vi "纳清DO电极校准.vi"() -> ()   [LabVIEW 2016, in "斯坦道多参数.lvlib"]
uses:
  <vilib>/Utility/miscctls.llb/LVPointTypeDef.ctl
  <vilib>/Analysis/NI_AALBase.lvlib
panel:
  out "标液2":string="饱和标准液"
  out "标液1":string="零点标准液"
  out "第二点信号值":dbl
  out "第一点信号值":dbl
  out "盐度":sgl format="%#.2f"
  out "大气压力":sgl format="%#.2f"
  out "饱和值":sgl format="%#.2f"
  out "报警信息":string
  out "通讯状态":string
  out "第二点校准值":dbl
  out "第一点校准值":dbl
  in  "校准停止":bool
  in  "校准启动":bool
  in  "校准模式":enum16{"两点校准", "单点校准"}(ring)=enum."单点校准"
  out "最小值":sgl format="%#.2f"
  out "最大值":sgl format="%#.2f"
  out "波形图表":sgl(graph) caption="历史曲线"
  out "mean":dbl caption="均值" format="%#.2f"
  out "standard deviation":dbl caption="标准差" format="%#.2f"
  out "变异系数":dbl format="%#.6f"
  out "测量值":sgl format="%#.2f"
  out "提示":string
  out "原始光强数值":sgl caption="信号值" format="%#.6f"
  out "温度":dbl format="%#.2f"
  # "DO电极设定"
  # "℃"
  # "mg/L"
  # "%"
  # "nA"
  # "kPa"
  # "ppt"
  # "请选择校准模式:"
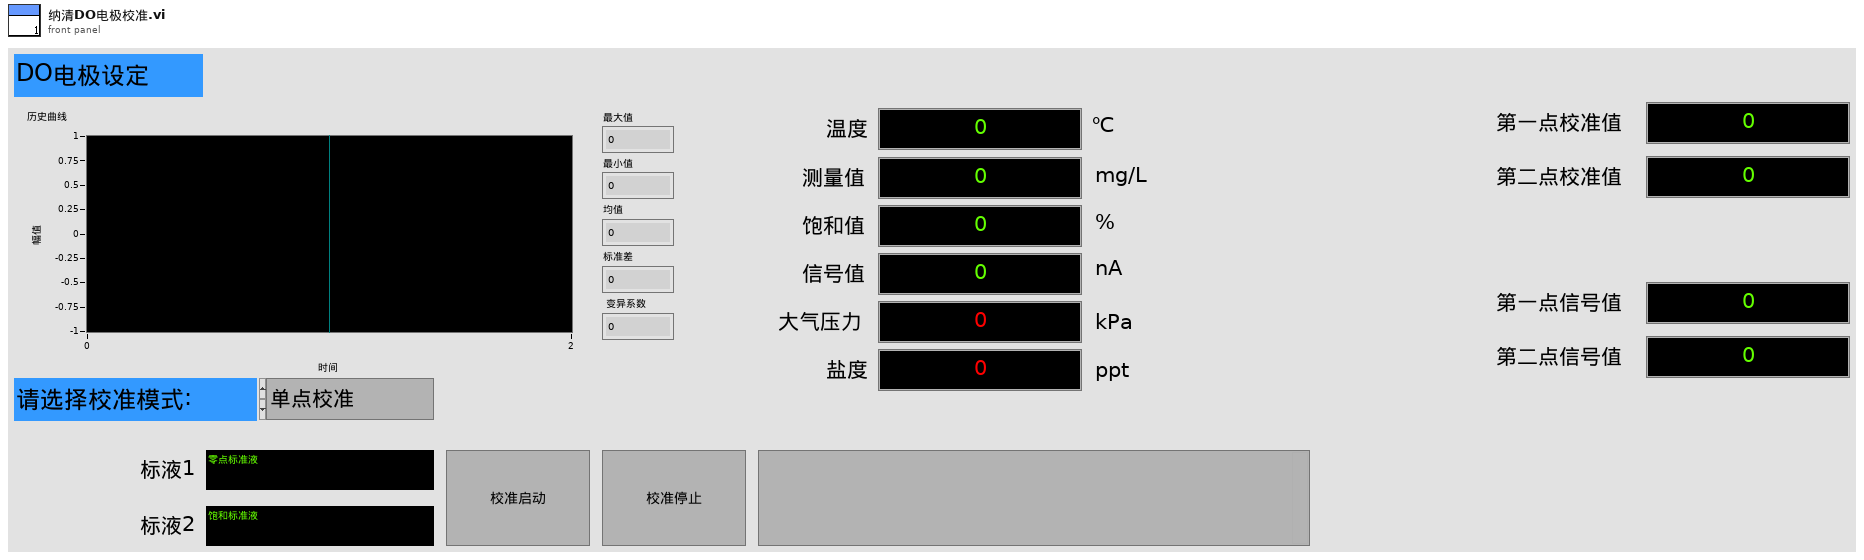
[diagram p1: front panel]
types:
  T1 = typedef "LVPointTypeDef.ctl" = cluster{"Horizontal":i16, "Vertical":i16}
  T2 = cluster{"报警码":u16, "溶解氧数值（mg/L）":sgl, "溶解氧数据（%）":sgl, "温度数据":sgl, "溶解氧原始信号 nA":sgl, "大气压力":sgl, "盐度":sgl, "0X0009_NC":string, "产品名称":string, "序列号":string, "硬件版本":string, "软件版本":string, "通讯地址":u16, "波特率":u16, "设备类型":u16, "0X0026_NC":string, "第一点原始数据":sgl, "第一点校准数据":sgl, "第二点原始数据":sgl, "第二点校准数据":sgl, "探头校准命令":u16, "温度校准参数":sgl, "温度校准命令":u16}
  T3 = enum8{"Enabled", "Disabled", "Disabled and Grayed Out"}
  T4 = cluster{"报警码":u16, "溶解氧数值（mg/L）":sgl, "溶解氧数据（%）":sgl, "温度数据":sgl, "溶解氧原始信号 nA":sgl, "大气压力":sgl, "盐度":sgl, "0X0009_NC":string, "产品名称":string, "序列号":string, "硬件版本":string, "软件版本":string, "通讯地址":u16, "波特率":u16, "设备类型":u16, "0X0026_NC":string, "第一点原始数据":sgl, "0X0033 NC":sgl, "第二点原始数据":sgl, "0X0037 NC":sgl, "探头校准命令":u16, "温度校准参数":sgl, "温度校准命令":u16}
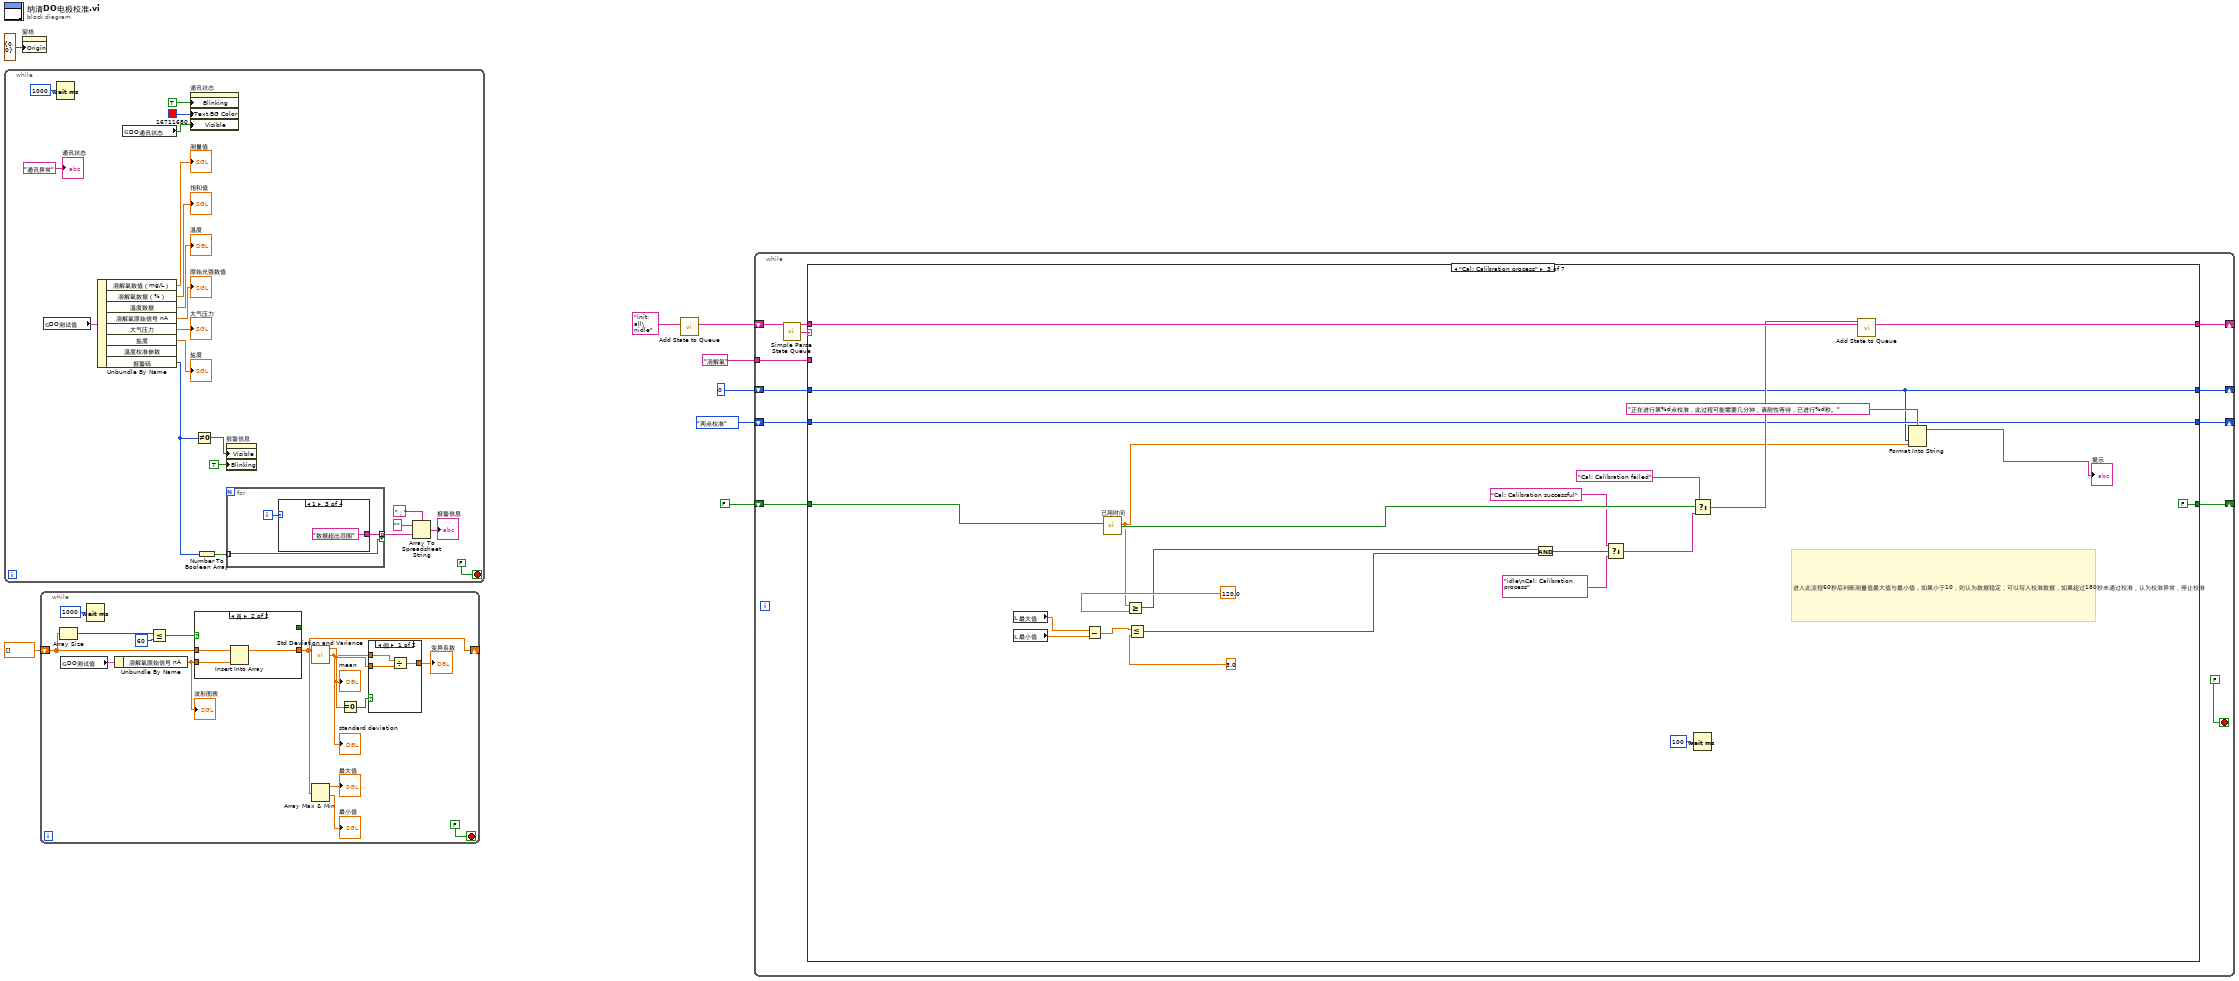
[diagram p0: block diagram]
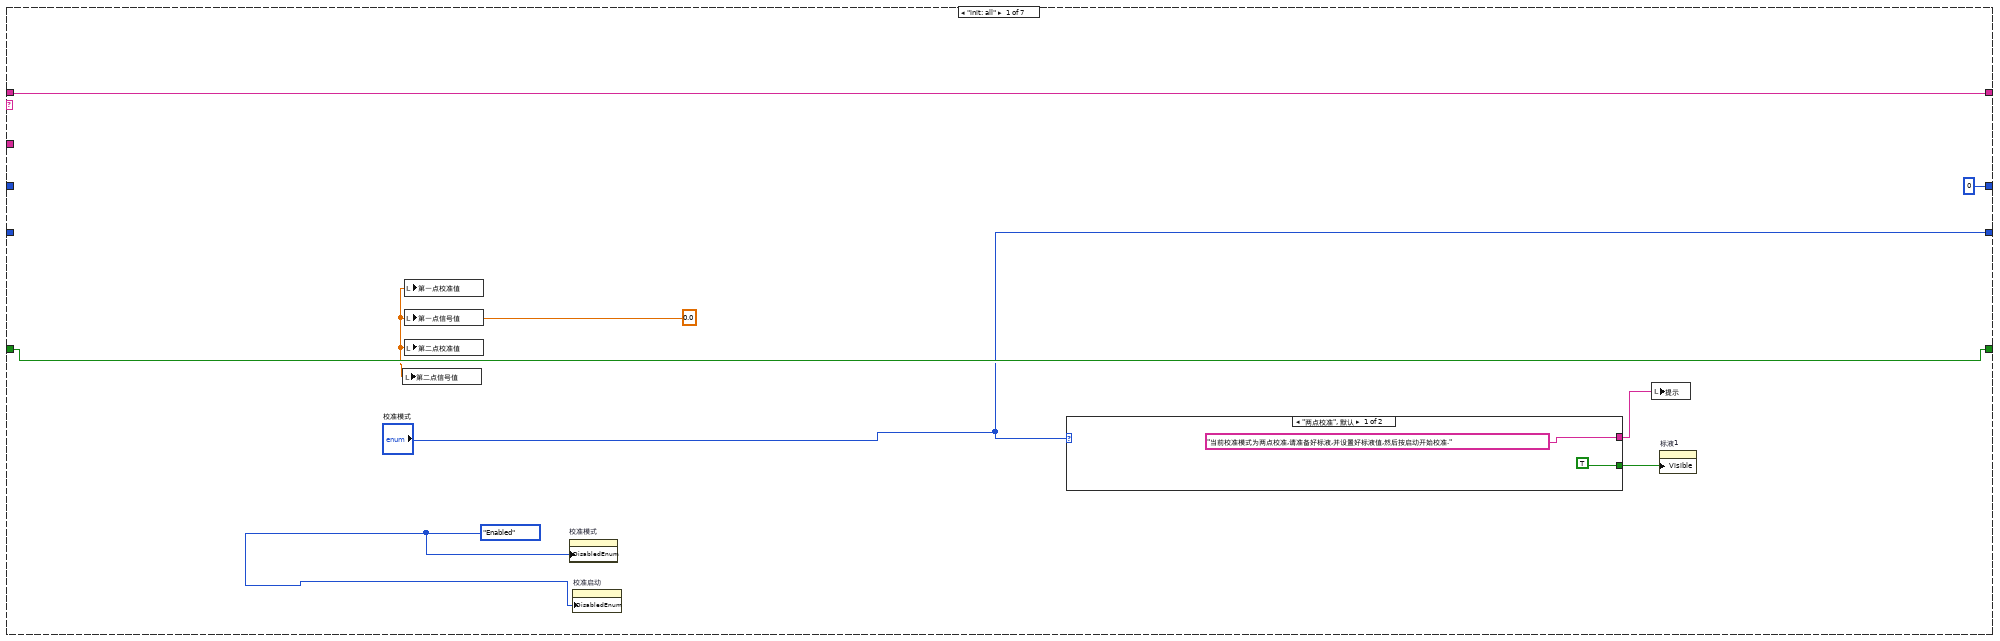
[diagram p2: hidden frame]
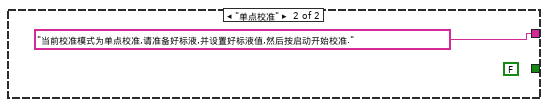
[diagram p3: hidden frame]
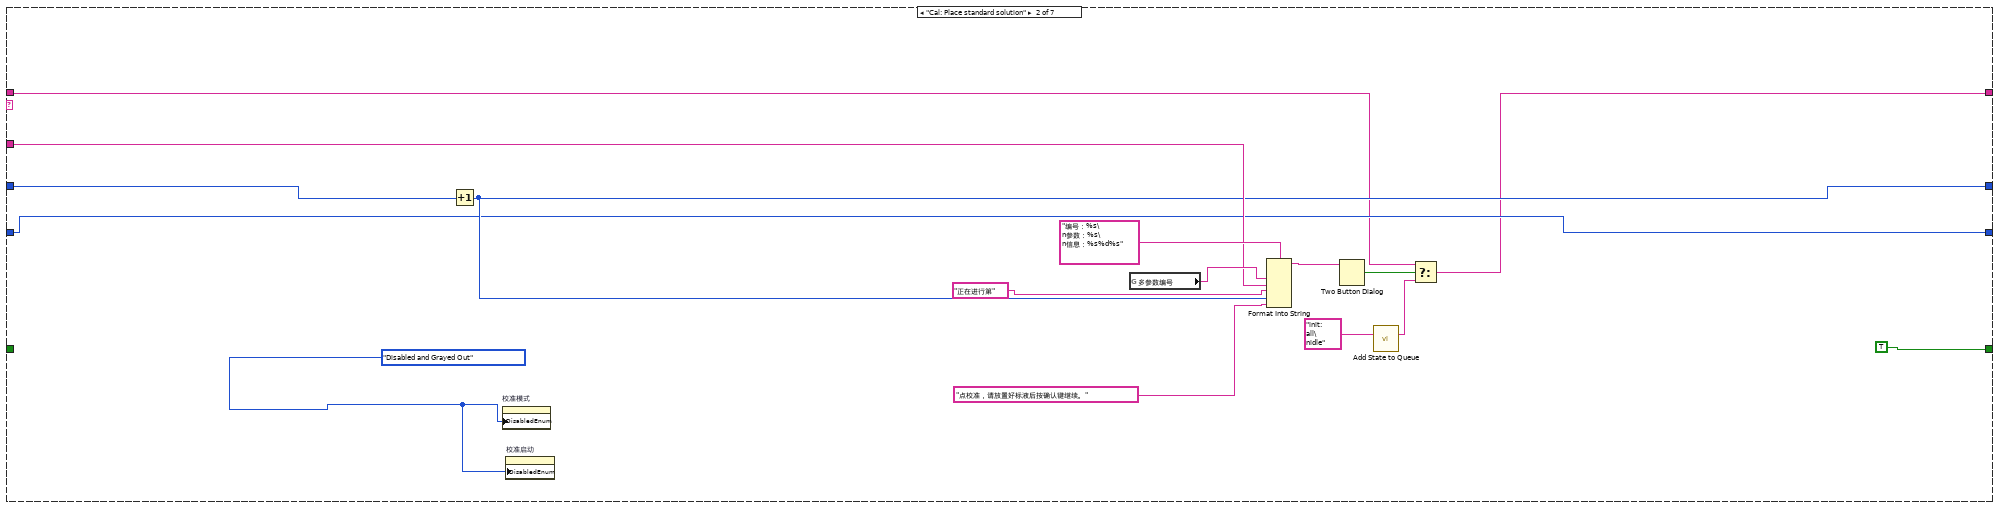
[diagram p4: hidden frame]
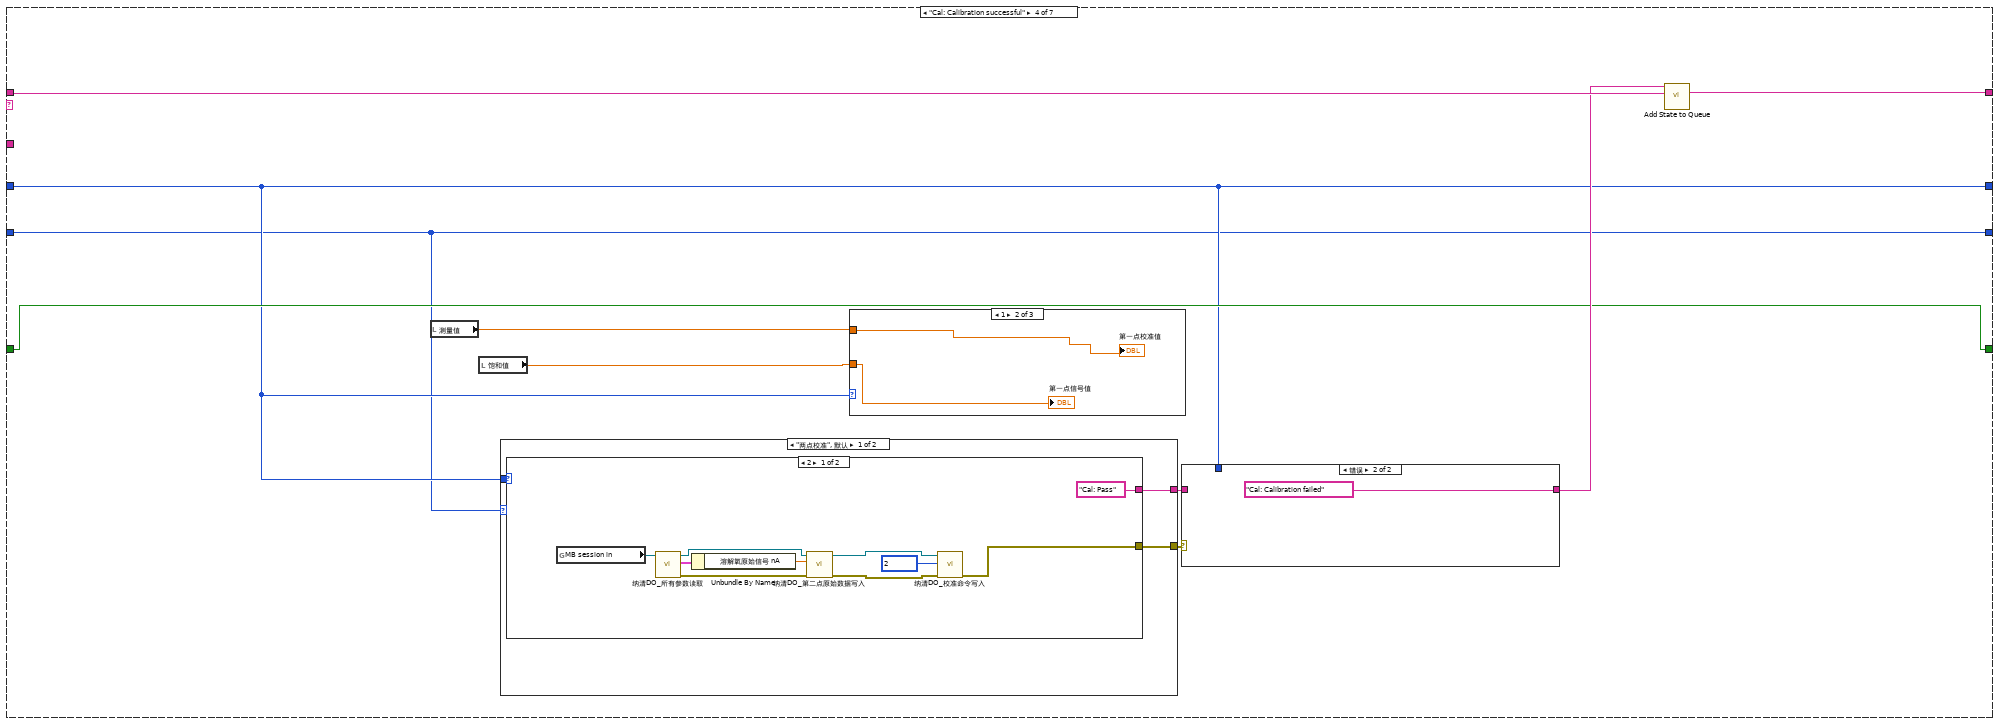
[diagram p5: hidden frame]
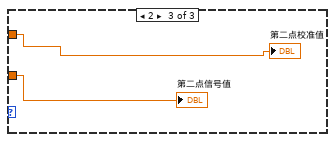
[diagram p7: hidden frame]
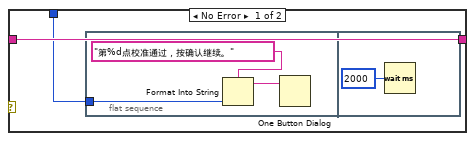
[diagram p8: hidden frame]
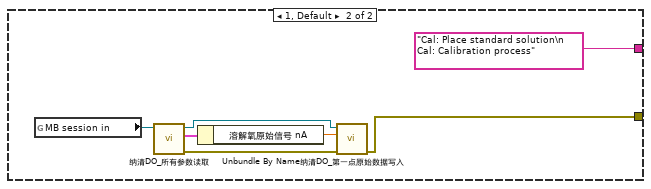
[diagram p9: hidden frame]
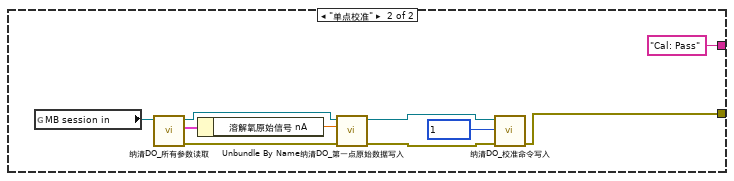
[diagram p10: hidden frame]
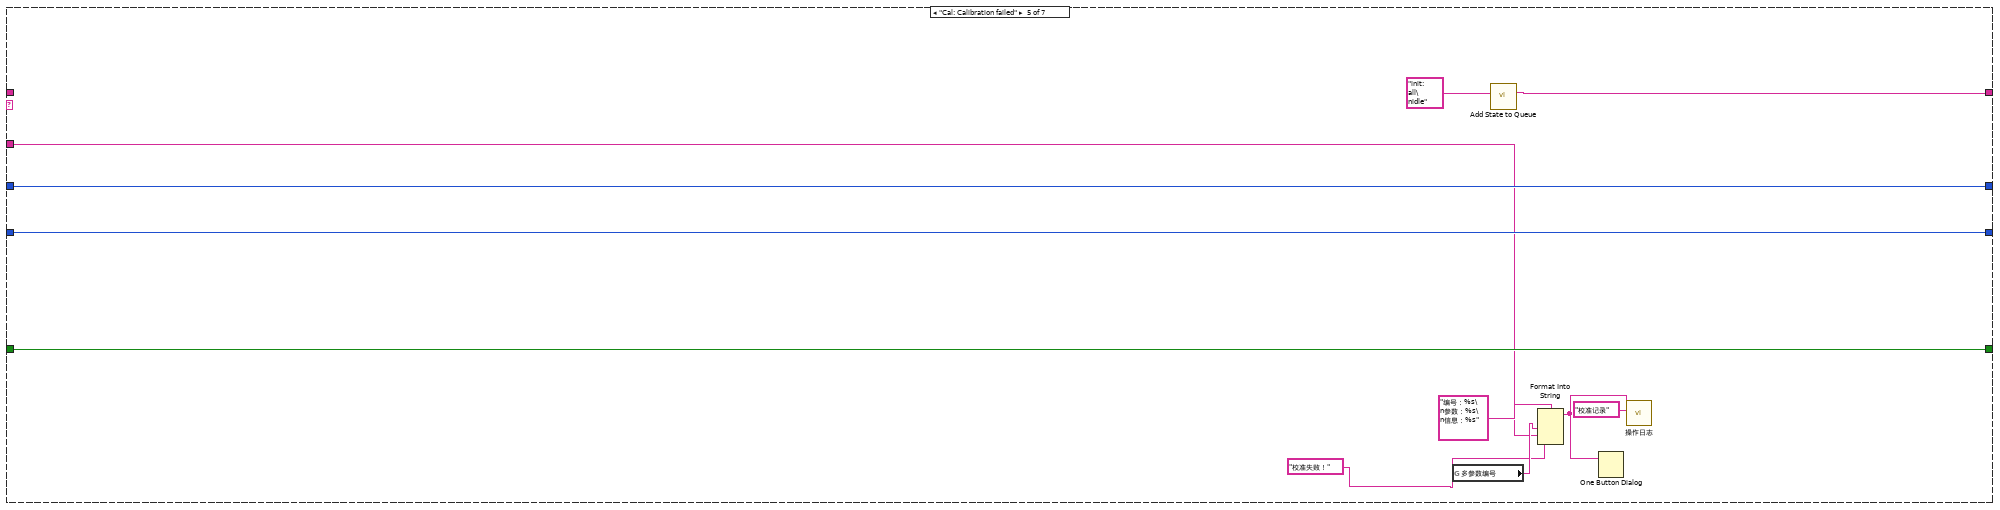
[diagram p11: hidden frame]
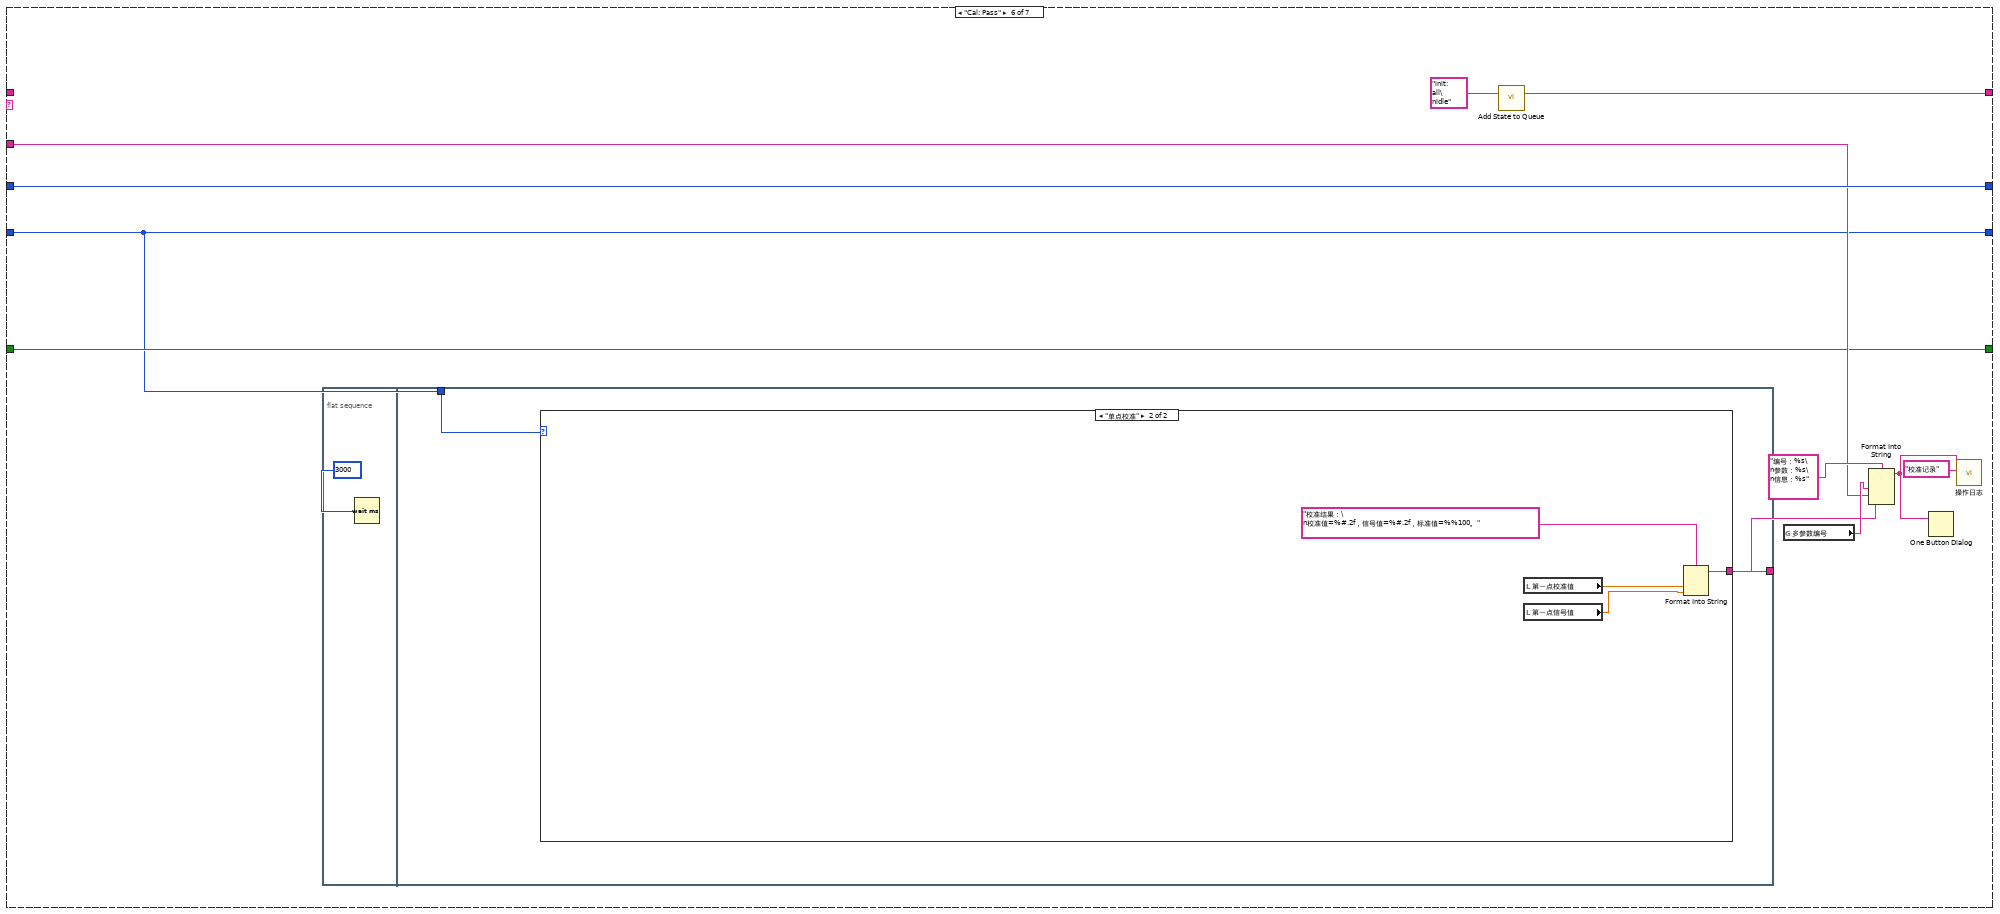
[diagram p12: hidden frame]
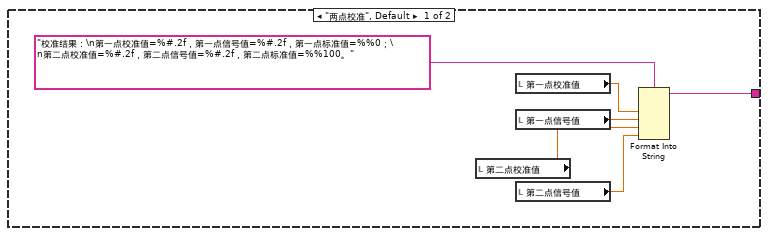
[diagram p13: hidden frame]
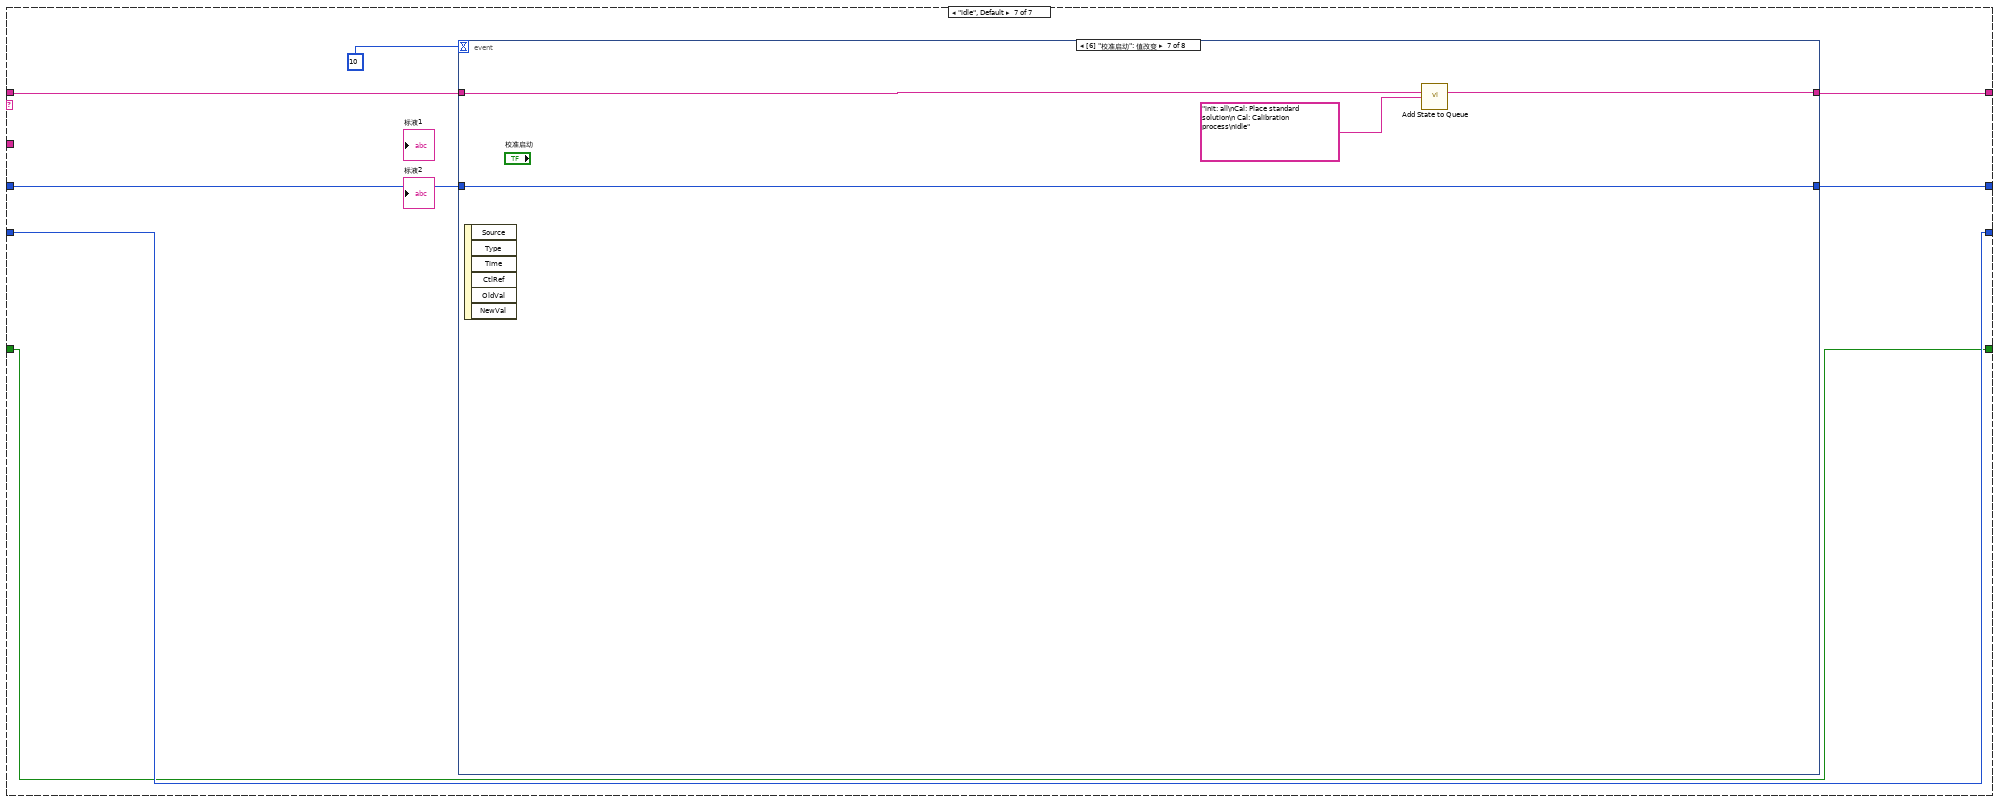
[diagram p14: hidden frame]
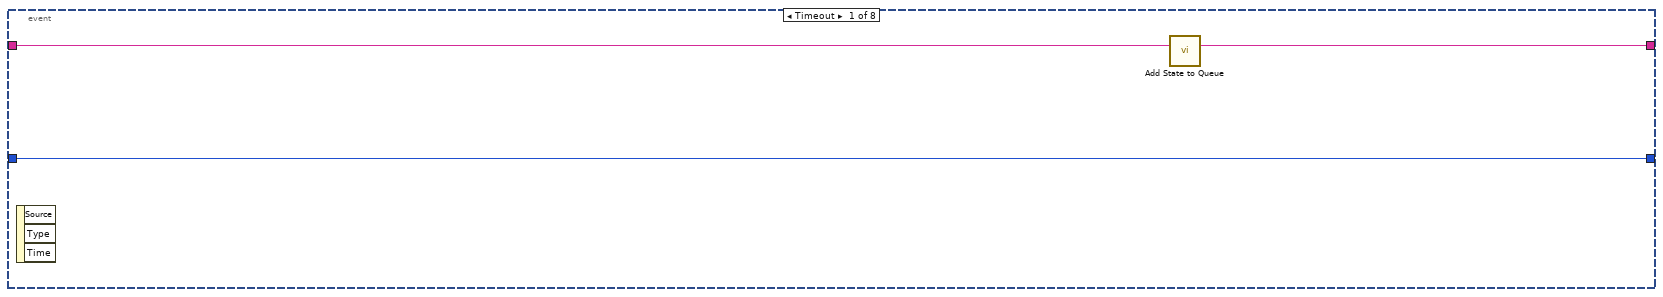
[diagram p15: hidden frame]
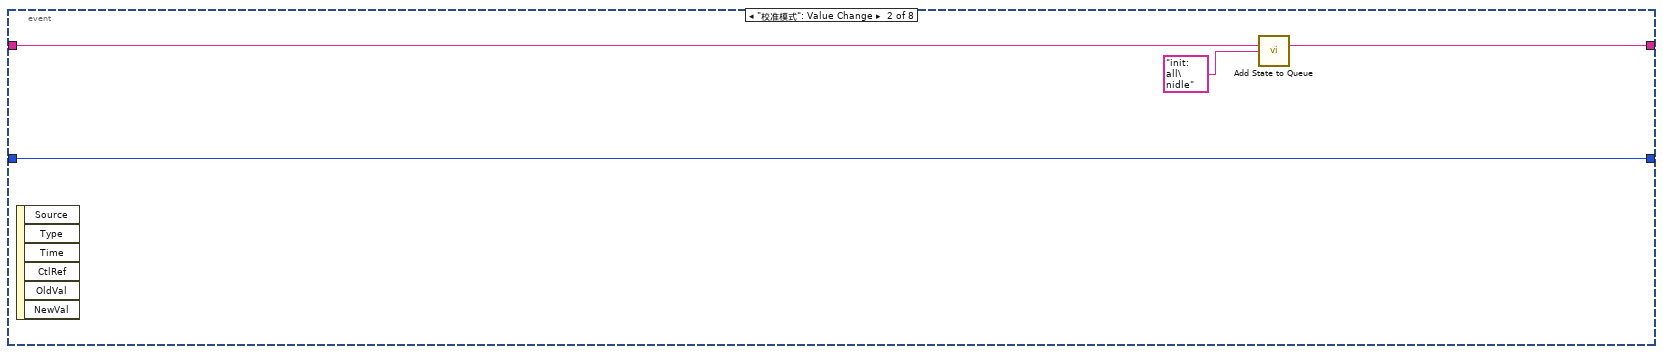
[diagram p16: hidden frame]
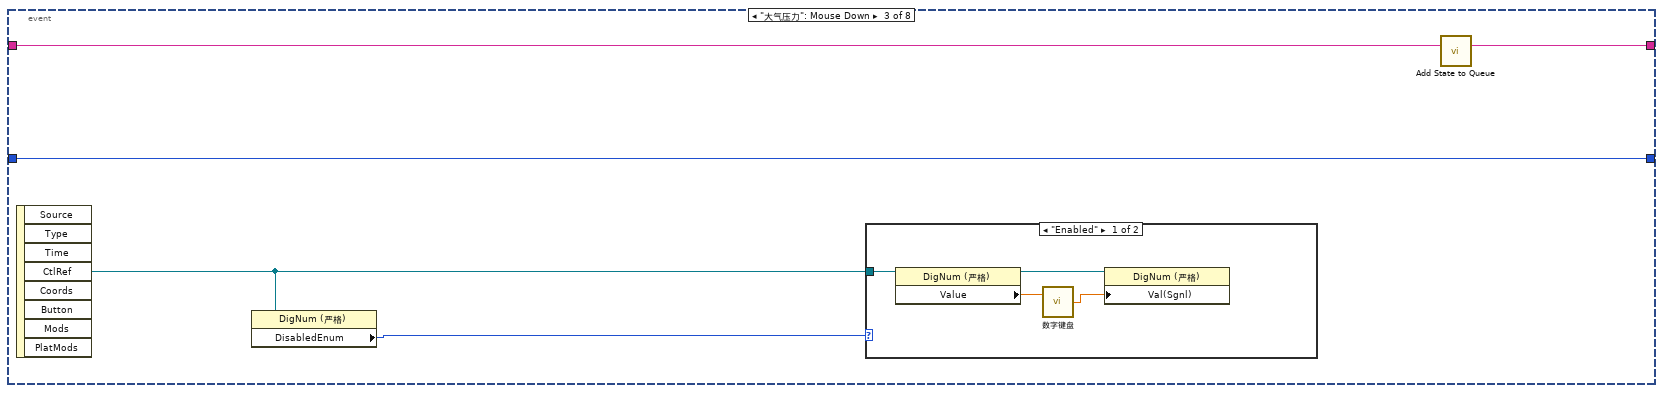
[diagram p17: hidden frame]
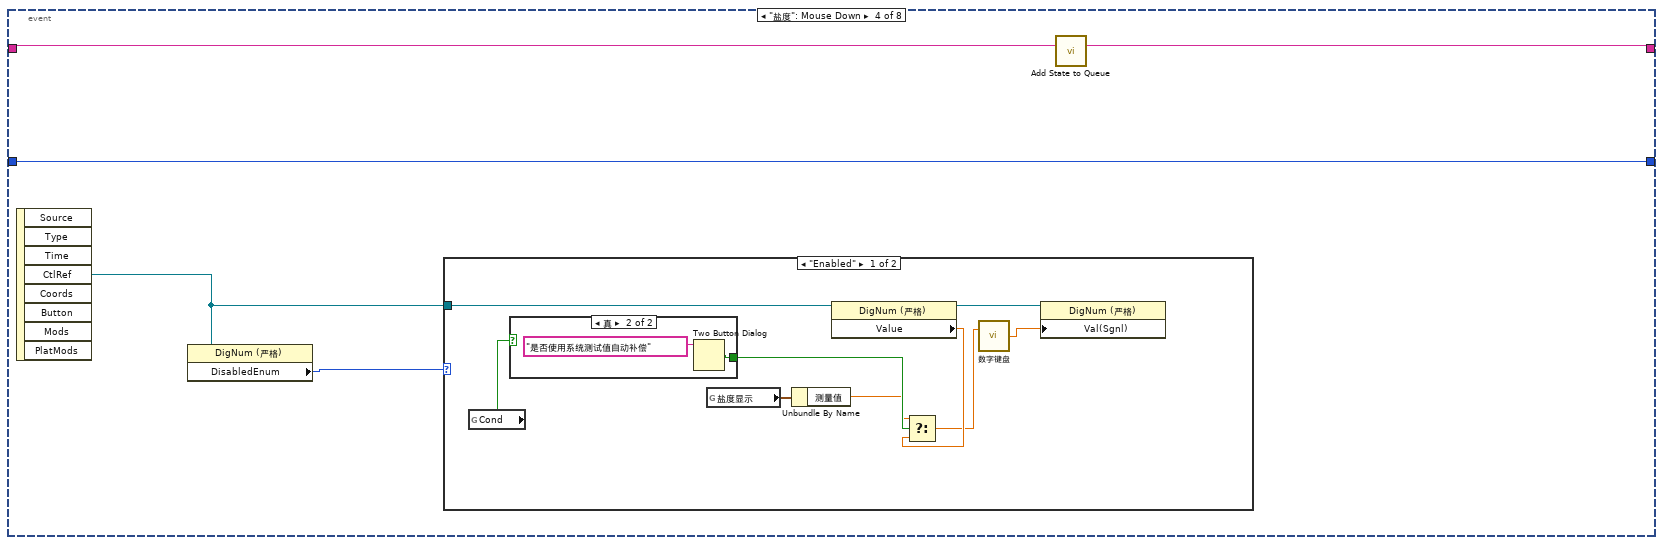
[diagram p19: hidden frame]
diagram:
  n1 = while {
    stop <- FALSE stop-if-true
    n2 = global read "纳清过程全局变量.vi" "DO测试值"() -> (w27:T2)
    n3 = Wait (ms)(milliseconds to wait=u32 1000 ("等待时间（毫秒）")) -> ()  [unwired: 1 out]
    n4 = Unbundle By Name(w27) -> ("溶解氧数值（mg/L）"=→"测量值":sgl, "溶解氧数据（%）"=→"饱和值":sgl, "温度数据"=→"温度":sgl, "溶解氧原始信号 nA"=→"原始光强数值":sgl, "大气压力"=→"大气压力":sgl, "盐度"=→"盐度":sgl, "报警码"=w14:u16)  [unwired: 1 out]
    n5 = global read "多参数全局变量.vi" "DO通讯状态"() -> (w20:bool)
    n6 = property on="通讯状态" class="Str"("Blinking"=TRUE ("闪烁"), "Text.BG Color"=u32 16711680, "Visible"=w20) -> ()  [unwired: 2 in, 2 out]
    n7 = Not Equal To 0?(x=w14) -> (x != 0?=w13:bool)
    n8 = Number To Boolean Array(number=w14) -> (Boolean array=w19:bool[])
    n9 = property on="报警信息" class="Str"("Visible"=w13, "Blinking"=TRUE ("闪烁")) -> ()  [unwired: 2 in, 2 out]
    n10 = for {
      tunnel: w19 -> [w30] mode=indexing
      tunnel: [w31] -> w18 mode=indexing if=w30
      i -> [w32]
      n11 = case shown="1" w32 {
        tunnel: [_ "温度超出范围" "数据超出范围" "温度传感器故障"] -> w31
        frame Default {
        }
        frame 0 {
        }
        frame 1 {
        }
        frame 8 {
        }
      }
    }
    n12 = Array To Spreadsheet String(delimiter (Tab)="；" ("分隔符(Tab)"), array=w18, 3:"" ("格式字符串")) -> (spreadsheet string=→"报警信息":string)
    "通讯状态" <- "通讯异常" ("当前串口")
  }
  n13 = property on="窗格" class="Pane"("Origin"=T1 {"Horizontal"=0, "Vertical"=0} ("原点")) -> ()  [unwired: 2 in, 2 out]
  n14 = while {
    shift-right: [w40] -> _
    shift-left: sgl[] [] -> [w46]
    stop <- FALSE stop-if-true
    n15 = Array Size(array=w46) -> (size(s)=w48:i32)
    n16 = global read "纳清过程全局变量.vi" "DO测试值"() -> (w36:T2)
    n17 = Wait (ms)(milliseconds to wait=u32 1000 ("等待时间（毫秒）")) -> ()  [unwired: 1 out]
    n18 = Unbundle By Name(w36) -> ("溶解氧原始信号 nA"=w37:sgl)
    "波形图表" <- w37
    n19 = Less Or Equal?(x=w48, y=60) -> (x <= y?=w47:bool)
    n20 = case shown="真" w47 {
      tunnel: w46 -> [w59 w62]
      tunnel: w37 -> [w57 w61]
      tunnel: [w55 w60] -> w40
      tunnel: [TRUE _] -> _
      frame False {
        n21 = Replace Array Subset(array=w59, new element=w57) -> (w58:sgl[])  [unwired: 1 in]
        n22 = Rotate 1D Array(1:w58, 2:-1 ("n")) -> (0:w55:sgl[])
      }
      frame True {
        n23 = Insert Into Array(array=w62, new element=w61) -> (w60:sgl[])  [unwired: 1 in]
      }
    }
    n24 = call <vilib>:"Std Deviation and Variance.vi"("X"=w40) -> ("mean"=w44:dbl, "standard deviation"=w43:dbl)  [unwired: 1 in, 1 out]
    "mean" <- w44
    "standard deviation" <- w43
    n25 = Array Max & Min(array=w40) -> (max value=→"最大值":sgl, min value=→"最小值":sgl)  [unwired: 2 out]
    n26 = Equal To 0?(x=w44) -> (x = 0?=w45:bool)
    n27 = case shown="假" w45 {
      tunnel: w43 -> [w53 _]
      tunnel: [w52 _] -> w42
      tunnel: w44 -> [w51 _]
      frame False {
        n28 = Divide(x=w53, y=w51) -> (x/y=w52:dbl)
      }
      frame True {
      }
    }
    "变异系数" <- w42
  }
  n29 = call "Add State to Queue.vi"("State(s) In (\"\")"="init: all\nidle" ("State(s) In (\"\")")) -> ("States Out"=w5:string)  [unwired: 14 in]
  n30 = while {
    shift-right: [w70] -> _
    shift-left: w5 -> [w74]
    shift-right: [w67] -> _
    shift-left: 0 -> [w69]
    tunnel: "溶解氧" ("State(s) In (\"\")") -> [w68]
    shift-right: [w65] -> _
    shift-left: enum16{"两点校准", "单点校准"}."两点校准" ("校准模式") -> [w66]
    shift-right: [w63] -> _
    shift-left: FALSE -> [w64]
    stop <- FALSE stop-if-true
    n31 = call "Simple Parse State Queue.vi"("State Queue"=w74) -> ("Remain States"=w71:string, "Next State"=w72:string)  [unwired: 13 in]
    n32 = case shown="\"Cal: Calibration process\"" w72 {
      tunnel: w71 -> [w82 w88 w120 w133 _ _ w218]
      tunnel: [w82 w87 w119 w132 w184 w188 w217] -> w70
      tunnel: w69 -> [_ w97 w104 w127 w187 w198 w215]
      tunnel: w68 -> [_ w98 _ _ w177 w194 _]
      tunnel: [0 w95 w104 w127 w187 w198 w216] -> w67
      tunnel: w66 -> [_ w94 w105 w126 w186 w190 w214]
      tunnel: ["校准模式" w94 w105 w126 w186 w190 w214] -> w65
      tunnel: w64 -> [w79 _ w107 w128 w185 w193 w212]
      tunnel: [w79 TRUE FALSE w128 w185 w193 w212] -> w63
      frame "init: all" {
        w76 = T3."Enabled" ("禁用")
        w78 = 0.0 ("第一点校准值")
        n33 = local write "第二点信号值"(w78) -> ()
        n34 = local write "第一点校准值"(w78) -> ()
        n35 = local write "第一点信号值"(w78) -> ()
        n36 = local write "第二点校准值"(w78) -> ()
        n37 = property on="校准模式" class="Enum (严格)"("DisabledEnum"=w76) -> ()  [unwired: 2 in, 2 out]
        n38 = property on="校准启动" class="Bool"("DisabledEnum"=w76) -> ()  [unwired: 2 in, 2 out]
        n39 = case shown="\"两点校准\", 默认" "校准模式" {
          tunnel: ["当前校准模式为两点校准,请准备好标液,并设置好标液值,然后按启动开始校准." ("提示") "当前校准模式为单点校准,请准备好标液,并设置好标液值,然后按启动开始校准." ("提示")] -> w81
          tunnel: [TRUE ("可见") _] -> w75
          frame "两点校准", Default {
          }
          frame "单点校准" {
            (unwired) FALSE ("可见")
          }
        }
        n40 = local write "提示"(w81) -> ()
        n41 = property on="标液1" class="Str"("Visible"=w75) -> ()  [unwired: 2 in, 2 out]
      }
      frame "Cal: Place standard solution" {
        w86 = T3."Disabled and Grayed Out" ("禁用")
        n42 = Increment(x=w97) -> (x+1=w95:i32)
        n43 = property on="校准模式" class="Enum (严格)"("DisabledEnum"=w86) -> ()  [unwired: 2 in, 2 out]
        n44 = property on="校准启动" class="Bool"("DisabledEnum"=w86) -> ()  [unwired: 2 in, 2 out]
        n45 = global read "多参数全局变量.vi" "多参数编号"() -> (w100:string)
        n46 = Format Into String(format string="编号：%s\n参数：%s\n信息：%s%d%s" ("格式字符串"), w100, w98, "正在进行第" ("消息"), w95, "点校准，请放置好标液后按确认键继续。" ("消息")) -> (resulting string=w92:string)  [unwired: 2 in, 1 out]
        n47 = Two Button Dialog(message=w92) -> (T button?=w91:bool)  [unwired: 2 in]
        n48 = call "Add State to Queue.vi"("State(s) In (\"\")"="init: all\nidle" ("State(s) In (\"\")")) -> ("States Out"=w89:string)  [unwired: 14 in]
        n49 = Select(t=w88, s=w91, f=w89) -> (s? t:f=w87:string)
      }
      frame "Cal: Calibration process" {
        # "进入此流程60秒后判断测量值最大值与最小值，如果小于10，则认为数据稳定，可以写入校准数据，如果超过180秒未通过校准，认为校准异常，停止校准"
        n50 = local read "最大值"() -> (w124:sgl)
        n51 = local read "最小值"() -> (w123:sgl)
        n52 = Subtract(x=w124, y=w123) -> (x-y=w125:sgl)
        n53 = call "已用时间"("Reset"=w107) -> ("Elapsed Time (s)"=w103:dbl, "Time has Elapsed"=w121:bool)  [unwired: 11 in, 6 out]
        n54 = Greater Or Equal?(x=w103, y=120.0) -> (x >= y?=w116:bool)
        n55 = Less Or Equal?(x=w125, y=3.0) -> (x <= y?=w112:bool)
        n56 = And(x=w116, y=w112) -> (x .and. y?=w113:bool)
        n57 = Select(t="Cal: Calibration successful" ("State(s) In (\"\")"), s=w113, f="idle\nCal: Calibration process" ("State(s) In (\"\")")) -> (s? t:f=w111:string)
        n58 = Wait (ms)(milliseconds to wait=u32 100 ("等待时间（毫秒）")) -> ()  [unwired: 1 out]
        n59 = Select(t="Cal: Calibration failed" ("State(s) In (\"\")"), s=w121, f=w111) -> (s? t:f=w110:string)
        n60 = call "Add State to Queue.vi"("State(s) In Front (\"\")"=w110, "State(s) In (\"\")"=w120) -> ("States Out"=w119:string)  [unwired: 13 in]
        n61 = Format Into String(format string="正在进行第%d点校准，此过程可能需要几分钟，请耐性等待，已进行%d秒。" ("格式字符串"), w104, w103) -> (resulting string=→"提示":string)  [unwired: 2 in, 1 out]
      }
      frame "Cal: Calibration successful" {
        n62 = local read "测量值"() -> (w129:sgl)
        n63 = local read "饱和值"() -> (w130:sgl)
        n64 = case shown="\"两点校准\", 默认" w126 {
          tunnel: [w149 w167] -> w135
          tunnel: [w148 "Cal: Pass" ("State(s) In (\"\")")] -> w134
          tunnel: w127 -> [w147 _]
          frame "两点校准", Default {
            n65 = case shown="2" w147 {
              tunnel: [w151 w160] -> w149
              tunnel: ["Cal: Pass" ("State(s) In (\"\")") "Cal: Place standard solution\n Cal: Calibration process" ("State(s) In (\"\")")] -> w148
              frame 2 {
                n66 = global read "多参数全局变量.vi" "MB session in"() -> (w156:refnum<class "MB_Master.lvclass">)
                n67 = call "纳清DO_所有参数读取.vi"("MB session in"=w156) -> ("error out"=w158:errorcluster, "输出值"=w155:T4, "MB session out"=w157:refnum<class "MB_Master.lvclass">)  [unwired: 8 in]
                n68 = Unbundle By Name(w155) -> ("溶解氧原始信号 nA"=w154:sgl)
                n69 = call "纳清DO_第二点原始数据写入.vi"("error in (no error)"=w158, "数值"=w154, "MB session in"=w157) -> ("error out"=w153:errorcluster, "MB session out"=w152:refnum<class "MB_Master.lvclass">)  [unwired: 7 in]
                n70 = call "纳清DO_校准命令写入.vi"("error in (no error)"=w153, "数值"=u16 2 ("starting address"), "MB session in"=w152) -> ("error out"=w151:errorcluster)  [unwired: 7 in, 1 out]
              }
              frame 1, Default {
                n71 = global read "多参数全局变量.vi" "MB session in"() -> (w163:refnum<class "MB_Master.lvclass">)
                n72 = call "纳清DO_所有参数读取.vi"("MB session in"=w163) -> ("error out"=w165:errorcluster, "输出值"=w162:T4, "MB session out"=w164:refnum<class "MB_Master.lvclass">)  [unwired: 8 in]
                n73 = Unbundle By Name(w162) -> ("溶解氧原始信号 nA"=w161:sgl)
                n74 = call "纳清DO_第一点原始数据写入.vi"("error in (no error)"=w165, "数值"=w161, "MB session in"=w164) -> ("error out"=w160:errorcluster)  [unwired: 7 in, 1 out]
              }
            }
          }
          frame "单点校准" {
            n75 = global read "多参数全局变量.vi" "MB session in"() -> (w173:refnum<class "MB_Master.lvclass">)
            n76 = call "纳清DO_所有参数读取.vi"("MB session in"=w173) -> ("error out"=w175:errorcluster, "输出值"=w172:T4, "MB session out"=w174:refnum<class "MB_Master.lvclass">)  [unwired: 8 in]
            n77 = Unbundle By Name(w172) -> ("溶解氧原始信号 nA"=w171:sgl)
            n78 = call "纳清DO_第一点原始数据写入.vi"("error in (no error)"=w175, "数值"=w171, "MB session in"=w174) -> ("error out"=w170:errorcluster, "MB session out"=w169:refnum<class "MB_Master.lvclass">)  [unwired: 7 in]
            n79 = call "纳清DO_校准命令写入.vi"("error in (no error)"=w170, "数值"=u16 1 ("starting address"), "MB session in"=w169) -> ("error out"=w167:errorcluster)  [unwired: 7 in, 1 out]
          }
        }
        n80 = case shown="1" w127 {
          tunnel: w130 -> [_ w137 w139]
          tunnel: w129 -> [_ w136 w138]
          frame 0, Default {
          }
          frame 1 {
            "第一点信号值" <- w137
            "第一点校准值" <- w136
          }
          frame 2 {
            "第二点信号值" <- w139
            "第二点校准值" <- w138
          }
        }
        n81 = case shown="错误" w135 {
          tunnel: w134 -> [w141 _]
          tunnel: [w141 "Cal: Calibration failed" ("State(s) In (\"\")")] -> w131
          tunnel: w127 -> [w140 _]
          frame No Error {
            n82 = flat-sequence {
              tunnel: w140 -> [w142]
              frame #0 {
                n83 = Format Into String(format string="第%d点校准通过，按确认继续。" ("格式字符串"), w142) -> (resulting string=w144:string)  [unwired: 2 in, 1 out]
                n84 = One Button Dialog(message=w144) -> ()  [unwired: 1 in, 1 out]
              }
              frame #1 {
                n85 = Wait (ms)(milliseconds to wait=u32 2000 ("等待时间（毫秒）")) -> ()  [unwired: 1 out]
              }
            }
          }
          frame Error {
          }
        }
        n86 = call "Add State to Queue.vi"("State(s) In Front (\"\")"=w131, "State(s) In (\"\")"=w133) -> ("States Out"=w132:string)  [unwired: 13 in]
      }
      frame "Cal: Calibration failed" {
        n87 = global read "多参数全局变量.vi" "多参数编号"() -> (w180:string)
        n88 = call "Add State to Queue.vi"("State(s) In (\"\")"="init: all\nidle" ("State(s) In (\"\")")) -> ("States Out"=w184:string)  [unwired: 14 in]
        n89 = Format Into String(format string="编号：%s\n参数：%s\n信息：%s" ("格式字符串"), w180, w177, "校准失败！" ("消息")) -> (resulting string=w179:string)  [unwired: 2 in, 1 out]
        n90 = One Button Dialog(message=w179) -> ()  [unwired: 1 in, 1 out]
        n91 = call "操作日志.vi"("table"="校准记录", "日志信息"=w179) -> ()  [unwired: 9 in, 1 out]
      }
      frame "Cal: Pass" {
        n92 = flat-sequence {
          tunnel: [w201] -> w191
          tunnel: w190 -> [w200]
          frame #0 {
            n93 = Wait (ms)(milliseconds to wait=u32 3000 ("等待时间（毫秒）")) -> ()  [unwired: 1 out]
          }
          frame #1 {
            n94 = case shown="\"单点校准\"" w200 {
              tunnel: [w207 w211] -> w201
              frame "两点校准", Default {
                n95 = local read "第二点校准值"() -> (w203:dbl)
                n96 = local read "第一点校准值"() -> (w205:dbl)
                n97 = local read "第一点信号值"() -> (w206:dbl)
                n98 = local read "第二点信号值"() -> (w202:dbl)
                n99 = Format Into String(format string="校准结果：\n第一点校准值=%#.2f，第一点信号值=%#.2f，第一点标准值=%%0；\n第二点校准值=%#.2f，第二点信号值=%#.2f，第二点标准值=%%100。" ("提示"), w205, w206, w203, w202) -> (resulting string=w207:string)  [unwired: 2 in, 1 out]
              }
              frame "单点校准" {
                n100 = local read "第一点校准值"() -> (w210:dbl)
                n101 = local read "第一点信号值"() -> (w208:dbl)
                n102 = Format Into String(format string="校准结果：\n校准值=%#.2f，信号值=%#.2f，标准值=%%100。" ("提示"), w210, w208) -> (resulting string=w211:string)  [unwired: 2 in, 1 out]
              }
            }
          }
        }
        n103 = call "Add State to Queue.vi"("State(s) In (\"\")"="init: all\nidle" ("State(s) In (\"\")")) -> ("States Out"=w188:string)  [unwired: 14 in]
        n104 = global read "多参数全局变量.vi" "多参数编号"() -> (w195:string)
        n105 = Format Into String(format string="编号：%s\n参数：%s\n信息：%s" ("格式字符串"), w195, w194, w191) -> (resulting string=w192:string)  [unwired: 2 in, 1 out]
        n106 = One Button Dialog(message=w192) -> ()  [unwired: 1 in, 1 out]
        n107 = call "操作日志.vi"("table"="校准记录", "日志信息"=w192) -> ()  [unwired: 9 in, 1 out]
      }
      frame "idle", Default {
        n108 = event shown="[6] \"校准启动\": 值改变" {
          selector: _ -> [_ _ _ _ _ _ _ _]
          dyn-events: _ -> [_ _ _ _ _ _ _ _]
          timeout: 10 -> [_ _ _ _ _ _ _ _]
          tunnel: w218 -> [w221 w225 w228 w235 w251 w256 w264 _]
          tunnel: [w220 w224 w229 w239 w255 w260 w263 w266] -> w217
          tunnel: [w219 w222 w230 w238 w254 w259 w261 w267] -> w216
          tunnel: w215 -> [w219 w222 w230 w238 w254 w259 w261 w267]
          event Timeout {
            n109 = event-data() -> ()  [unwired: 1 in, 3 out]
            n110 = call "Add State to Queue.vi"("State(s) In (\"\")"=w221) -> ("States Out"=w220:string)  [unwired: 14 in]
          }
          event "校准模式": Value Change {
            n111 = event-data() -> ()  [unwired: 1 in, 6 out]
            n112 = call "Add State to Queue.vi"("State(s) In (\"\")"=w225, "State(s) At Back (\"\")"="init: all\nidle" ("State(s) In (\"\")")) -> ("States Out"=w224:string)  [unwired: 13 in]
          }
          event "大气压力": Mouse Down {
            n113 = event-data() -> ("CtlRef"=w227:refnum<vi>)  [unwired: 1 in, 7 out]
            n114 = property class="DigNum (严格)"(reference=w227) -> ("DisabledEnum"=w226:T3)  [unwired: 1 in, 2 out]
            n115 = case shown="\"Enabled\"" w226 {
              tunnel: w227 -> [w234 _]
              frame "Enabled" {
                n116 = property class="DigNum (严格)"(reference=w234) -> (reference out=w231:refnum<vi>, "Value"=w232:sgl)  [unwired: 1 in, 1 out]
                n117 = call "数字键盘.vi"("OldNumber"=w232) -> ("NewNumber"=w233:dbl)  [unwired: 1 in]
                n118 = property class="DigNum (严格)"(reference=w231, "Val(Sgnl)"=w233) -> ()  [unwired: 1 in, 2 out]
              }
              frame "Disabled", Default {
              }
            }
            n119 = call "Add State to Queue.vi"("State(s) In (\"\")"=w228) -> ("States Out"=w229:string)  [unwired: 14 in]
          }
          event "盐度": Mouse Down {
            n120 = event-data() -> ("CtlRef"=w236:refnum<vi>)  [unwired: 1 in, 7 out]
            n121 = property class="DigNum (严格)"(reference=w236) -> ("DisabledEnum"=w237:T3)  [unwired: 1 in, 2 out]
            n122 = case shown="\"Enabled\"" w237 {
              tunnel: w236 -> [w248 _]
              frame "Enabled" {
                n123 = global read "断电保存变量.vi" "Cond"() -> (w240:bool)
                n124 = case shown="真" w240 {
                  tunnel: [_ w249] -> w245
                  frame False {
                  }
                  frame True {
                    n125 = Two Button Dialog(message="是否使用系统测试值自动补偿" ("消息")) -> (T button?=w249:bool)  [unwired: 2 in]
                  }
                }
                n126 = global read "多参数全局变量.vi" "盐度显示"() -> (w244:cluster{"温度测量值":sgl, "测量值":sgl, "温度偏移修正值":sgl})
                n127 = Unbundle By Name(w244) -> ("测量值"=w243:sgl)
                n128 = property class="DigNum (严格)"(reference=w248) -> (reference out=w246:refnum<vi>, "Value"=w242:sgl)  [unwired: 1 in, 1 out]
                n129 = Select(t=w243, s=w245, f=w242) -> (s? t:f=w241:sgl)
                n130 = call "数字键盘.vi"("OldNumber"=w241) -> ("NewNumber"=w247:dbl)  [unwired: 1 in]
                n131 = property class="DigNum (严格)"(reference=w246, "Val(Sgnl)"=w247) -> ()  [unwired: 1 in, 2 out]
              }
              frame "Disabled", Default {
              }
            }
            n132 = call "Add State to Queue.vi"("State(s) In (\"\")"=w235) -> ("States Out"=w239:string)  [unwired: 14 in]
          }
          event "大气压力": Value Change {
            n133 = event-data() -> ("NewVal"=w252:sgl)  [unwired: 1 in, 3 out]
            n134 = global read "多参数全局变量.vi" "MB session in"() -> (w253:refnum<class "MB_Master.lvclass">)
            n135 = call "纳清DO_大气压力写入.vi"("数值"=w252, "MB session in"=w253) -> ()  [unwired: 8 in, 2 out]
            n136 = call "Add State to Queue.vi"("State(s) In (\"\")"=w251) -> ("States Out"=w255:string)  [unwired: 14 in]
          }
          event "盐度": Value Change {
            n137 = event-data() -> ("NewVal"=w257:sgl)  [unwired: 1 in, 5 out]
            n138 = global read "多参数全局变量.vi" "MB session in"() -> (w258:refnum<class "MB_Master.lvclass">)
            n139 = call "纳清DO_盐度写入.vi"("数值"=w257, "MB session in"=w258) -> ()  [unwired: 8 in, 2 out]
            n140 = call "Add State to Queue.vi"("State(s) In (\"\")"=w256) -> ("States Out"=w260:string)  [unwired: 14 in]
          }
          event "校准启动": Value Change {
            n141 = event-data() -> ()  [unwired: 1 in, 6 out]
            n142 = call "Add State to Queue.vi"("State(s) In (\"\")"=w264, "State(s) At Back (\"\")"="init: all\nCal: Place standard solution\n Cal: Calibration process\nidle" ("State(s) In (\"\")")) -> ("States Out"=w263:string)  [unwired: 13 in]
          }
          event "校准停止": Value Change {
            n143 = event-data() -> ()  [unwired: 1 in, 6 out]
            n144 = call "Add State to Queue.vi"("State(s) In (\"\")"="init: all\nidle" ("State(s) In (\"\")")) -> ("States Out"=w266:string)  [unwired: 14 in]
          }
        }
      }
    }
  }
